vi "Add Menu Items.vi"(7 "Menu control":enum16{"Pulse", "Post-process", "Monitor"}(ring), 8 "error in (no error)":errorcluster, 9 "Reset":bool, 10 "Item Names":string[](array[string]), 11 "Monitor-Pulse in":refnum<class "Monitor-Pulse.lvclass">) -> (0 "error out":errorcluster, 3 "Monitor-Pulse out":refnum<class "Monitor-Pulse.lvclass">)   [LabVIEW 2015, in "Monitor-Pulse.lvclass"]
uses:
  Monitor-Pulse.lvclass
  Monitor-Pulse.lvclass/Monitor-Pulse.ctl
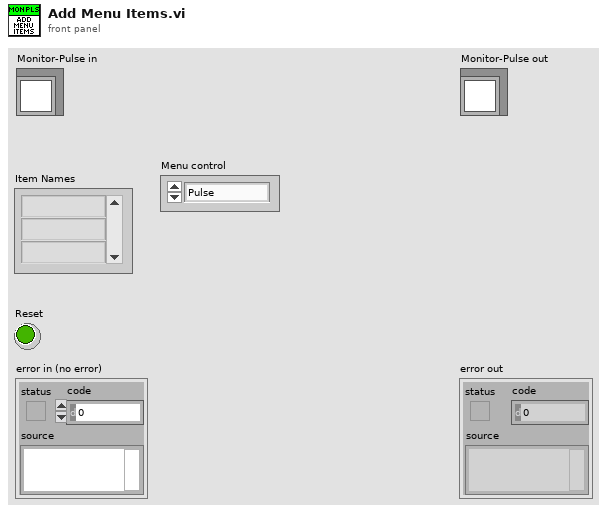
[diagram p1: front panel]
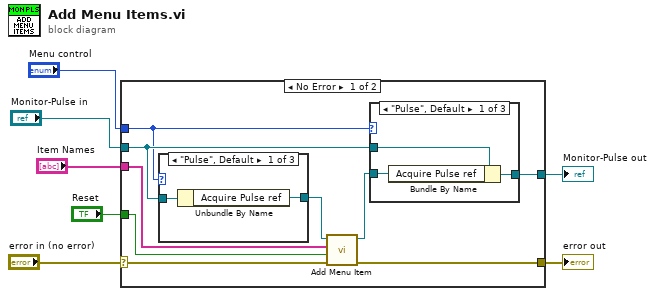
[diagram p0: block diagram]
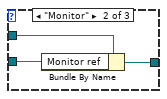
[diagram p2: hidden frame]
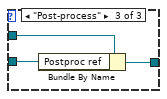
[diagram p3: hidden frame]
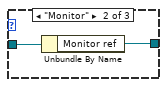
[diagram p4: hidden frame]
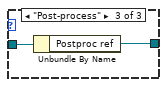
[diagram p5: hidden frame]
diagram:
  n1 = case shown="No Error" "error in (no error)" {
    selector: "error in (no error)" -> [w11 w33]
    tunnel: [w13 w33] -> w6
    tunnel: [w12 w32] -> w4
    tunnel: "Monitor-Pulse in" -> [w15 w32]
    tunnel: "Item Names" -> [w10 _]
    tunnel: "Reset" -> [w9 _]
    tunnel: "Menu control" -> [w8 _]
    frame No Error {
      n2 = case shown="\"Pulse\", Default" w8 {
        tunnel: [w27 w29 w31] -> w16
        tunnel: w15 -> [w26 w28 w30]
        frame "Pulse", Default {
          n3 = Unbundle By Name(w26) -> ("Acquire Pulse ref"=w27:refnum<vi>)
        }
        frame "Monitor" {
          n4 = Unbundle By Name(w28) -> ("Monitor ref"=w29:refnum<vi>)
        }
        frame "Post-process" {
          n5 = Unbundle By Name(w30) -> ("Postproc ref"=w31:refnum<vi>)
        }
      }
      n6 = call "Add Menu Item.vi"("error in (no error)"=w11, "Reset"=w9, "Item Names"=w10, "Queed Listbox ref"=w16) -> ("error out"=w13:errorcluster, "Queed Listbox ref out"=w14:refnum<vi>)  [unwired: 5 in, 1 out]
      n7 = case shown="\"Pulse\", Default" w8 {
        tunnel: w15 -> [w19 w22 w25]
        tunnel: w14 -> [w18 w21 w24]
        tunnel: [w17 w20 w23] -> w12
        frame "Pulse", Default {
          n8 = Bundle By Name(cluster=w19, "Acquire Pulse ref"=w18) -> (w17:refnum<class "Monitor-Pulse.lvclass">)
        }
        frame "Monitor" {
          n9 = Bundle By Name(cluster=w22, "Monitor ref"=w21) -> (w20:refnum<class "Monitor-Pulse.lvclass">)
        }
        frame "Post-process" {
          n10 = Bundle By Name(cluster=w25, "Postproc ref"=w24) -> (w23:refnum<class "Monitor-Pulse.lvclass">)
        }
      }
    }
    frame Error {
    }
  }
  "error out" <- w6
  "Monitor-Pulse out" <- w4
